vi "Default Configuration.vi"() -> (3 "Default Configuration":T1={"Common"={"Period (s)"=0.001, "Offset (us)"=0, "ClockID"=0, "Priority"=100, "Processor"=-2}, "Step"=100} {"Common"."Period (s)" format="%#_13g"})   [LabVIEW 2021, in "TemplatePlugin.lvclass"]
uses:
  TemplatePlugin.lvclass
  Common/Typedef/Configuration.ctl
  CIF-LVCore/src/CIFCore/Common/Typedef/Common Plugin Configuration.ctl
  CIF-LVCore/src/CIFCore/Common/CIFCoreCommon.lvlib
  Common/TemplateCommon.lvlib
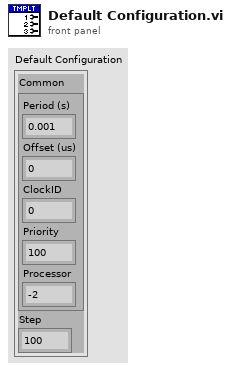
[diagram p1: front panel]
types:
  T1 = typedef "TemplateCommon.lvlib/Configuration.ctl" = cluster{"Common":T2, "Step":u64}
  T2 = typedef "CIFCoreCommon.lvlib/Common Plugin Configuration.ctl" = cluster{"Period (s)":dbl, "Offset (us)":i32, "ClockID":u8, "Priority":i32, "Processor":i32}
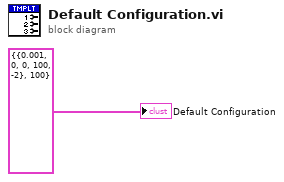
[diagram p0: block diagram]
diagram:
  "Default Configuration" <- T1 {"Common"={"Period (s)"=0.001, "Offset (us)"=0, "ClockID"=0, "Priority"=100, "Processor"=-2}, "Step"=100} ("Template Configuration")
